vi "Tosca-Enqueue Output State.vi"(0 "State":refnum<class "State.lvclass">, 2 "IPC":T1, 5 "AODO":T2, 11 "error in":errorcluster) -> (4 "State out":refnum<class "State.lvclass">, 15 "error out":errorcluster)   [LabVIEW 2020]
uses:
  Typedefs/Tosca-State AODO.ctl
  epl-vi-lib/Signal Synthesis VIs/4th Generation/Classes/SignalManager/SignalManager.lvclass
  Typedefs/Tosca-AO Runtime.ctl
  Typedefs/Tosca-DO Runtime.ctl
  IPC VIs/Tosca-IPC.ctl
  Classes/Parameters/Parameters.lvclass
  Digital Input VIs/Tosca-DI Queue Data.ctl
  Digital Input VIs/Tosca-Input Event.ctl
  Digital Input VIs/Tosca-Input Criterion.ctl
  epl-vi-lib/Utility VIs/Type Defs/Logic State.ctl
  Typedefs/Tosca-Accumulator.ctl
  Typedefs/Tosca-Synapse Start Data.ctl
  IPC VIs/Tosca-Message.ctl
  IPC VIs/Tosca-Message Action.ctl
  Typedefs/Tosca-Thread Type.ctl
  Imaging VIs/Tosca-2P-Notifier Data.ctl
  Typedefs/Tosca-MATLAB Queue Data.ctl
  Visual Stim VIs/Tosca-Grating.ctl
  Visual Stim VIs/Tosca-Grating Type.ctl
  Typedefs/Tosca-File IO Notification.ctl
  Classes/State/State.lvclass
  Classes/State/State.lvclass/State.ctl
  Trace VIs/Tosca-Trace-Event.ctl
  Classes/State/Read Grating.vi
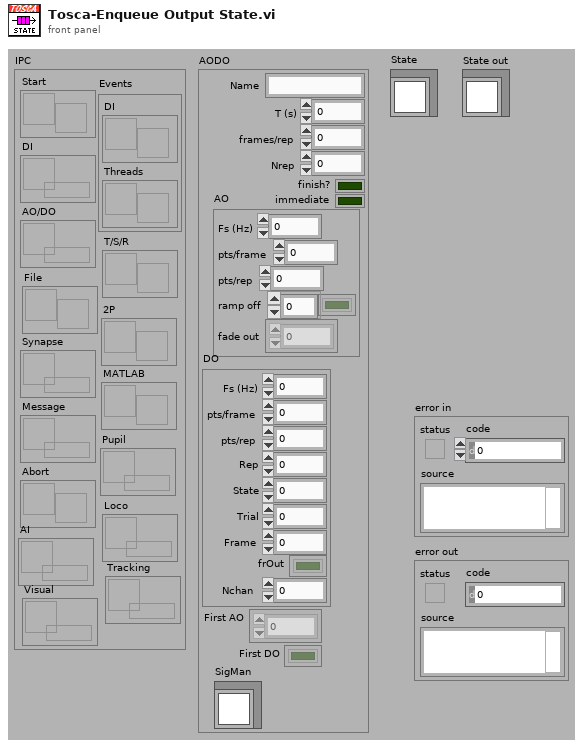
[diagram p1: front panel]
types:
  T1 = typedef "Tosca-IPC.ctl" = cluster{"Start":refnum<notifier>, "DI":refnum<queue>, "AO/DO":refnum<queue>, "Synapse":refnum<queue>, "Message":refnum<queue>, "Abort":refnum<notifier>, "Events":cluster{"DI":refnum<user-event>, "Threads ":refnum<user-event>}, "T/S/R":refnum<notifier>, "2P":refnum<notifier>, "MATLAB":refnum<notifier>, "Pupil":refnum<queue>, "Loco":refnum<queue>, "AI":refnum<queue>, "Tracking":refnum<queue>, "Visual":refnum<queue>, "File":refnum<notifier>}
  T2 = typedef "Tosca-State AODO.ctl" = cluster{"Name":string, "T (s)":dbl, "First AO":dbl[][], "frames/rep":i32, "finish?":bool, "Nrep":i32, "AO":T3, "DO":T4, "immediate":bool, "First DO":bool[][], "SigMan":refnum<class "SignalManager.lvclass">}
  T3 = typedef "Tosca-AO Runtime.ctl" = cluster{"Fs (Hz)":dbl, "pts/frame":i32, "pts/rep":i32, "ramp off":bool[], "fade out":dbl[][]}
  T4 = typedef "Tosca-DO Runtime.ctl" = cluster{"Fs (Hz)":dbl, "pts/frame":i32, "pts/rep":i32, "Rep":i32, "State":i32, "Trial":i32, "Frame":i32, "frOut":bool[], "Nchan":i32}
  T5 = typedef "Tosca-Grating Type.ctl" = enum16{"OFF", "Square", "Sine"}
  T6 = typedef "Tosca-Trace-Event.ctl" = enum16{"Unspecified", "Trial start", "Enqueue", "Result", "End parser", "Frame", "Queue available", "Timeout sent", "WritePos", "TTL"}
  T7 = typedef "Tosca-Grating.ctl" = cluster{"Type":T5, "Orientation (deg)":dbl, "Spatial frequency (cpd)":dbl, "Velocity (Hz)":dbl, "Contrast":dbl, "Background intensity":dbl, "Duration (ms)":dbl, "Phase (cycles)":dbl}
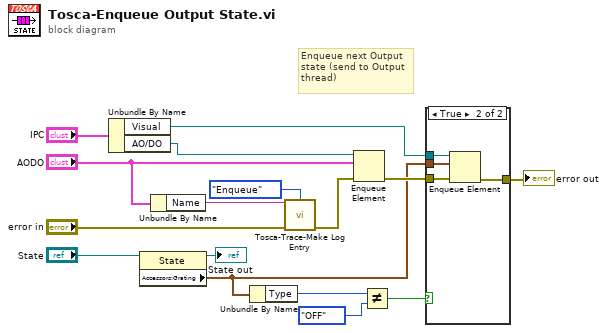
[diagram p0: block diagram]
diagram:
  # "Enqueue next Output state (send to Output thread)"
  n1 = Unbundle By Name("IPC") -> ("Visual"=w8:refnum<queue>, "AO/DO"=w12:refnum<queue>)
  n2 = property class="State"(reference="State") -> (reference out=→"State out":refnum<class "State.lvclass">, "Accessors:Grating"=w4:T7)  [unwired: 1 in, 1 out]
  n3 = Unbundle By Name("AODO") -> ("Name"=w16:string)
  n4 = Unbundle By Name(w4) -> ("Type"=w3:T5)
  n5 = call "Tosca-Trace-Make Log Entry.vi"("Message"=w16, "Event"=Tosca-Trace-Event."Enqueue", "error in (no error)"="error in") -> ("error out"=w13:errorcluster)  [unwired: 12 in]
  n6 = Enqueue Element(queue=w12, element="AODO", error in (no error)=w13) -> (error out=w9:errorcluster)  [unwired: 1 in, 2 out]
  n7 = Not Equal?(x=w3, y=Tosca-Grating_Type."OFF") -> (x != y?=w6:bool)
  n8 = case shown="True" w6 {
    tunnel: w9 -> [w17 w21]
    tunnel: w8 -> [_ w20]
    tunnel: [w17 w19] -> w7
    tunnel: w4 -> [_ w18]
    frame False {
    }
    frame True {
      n9 = Enqueue Element(queue=w20, element=w18, error in (no error)=w21) -> (error out=w19:errorcluster)  [unwired: 1 in, 2 out]
    }
  }
  "error out" <- w7
